vi "Write Create Tags_.vi"(8 "error in (no error)":errorcluster, 10 "Create Tags?":bool=TRUE, 11 "CVT configuration in":refnum<class "CVT configuration.lvclass">) -> (0 "error out":errorcluster, 3 "CVT configuration out":refnum<class "CVT configuration.lvclass">)   [LabVIEW 2013, in "CVT configuration.lvclass"]
uses:
  CVT configuration.lvclass
  CVT configuration.lvclass/CVT configuration.ctl
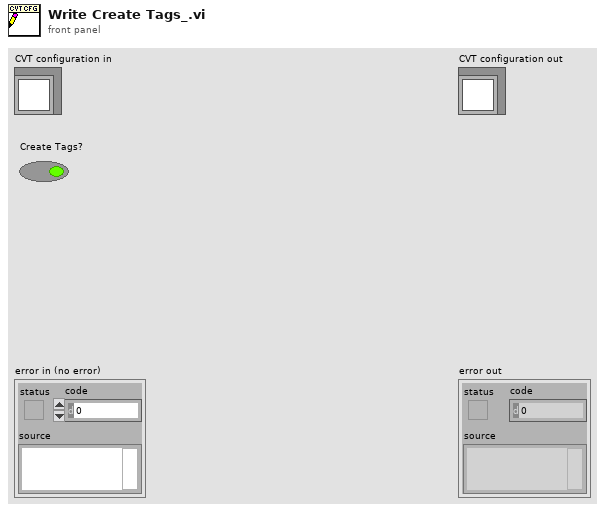
[diagram p1: front panel]
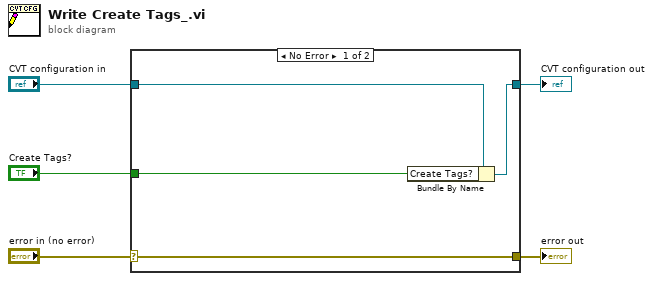
[diagram p0: block diagram]
diagram:
  n1 = case shown="No Error" "error in (no error)" {
    selector: "error in (no error)" -> [w9 w10]
    tunnel: [w9 w10] -> w4
    tunnel: [w7 w11] -> w2
    tunnel: "CVT configuration in" -> [w8 w11]
    tunnel: "Create Tags?" -> [w6 _]
    frame No Error {
      n2 = Bundle By Name(cluster=w8, "Create Tags?"=w6) -> (w7:refnum<class "CVT configuration.lvclass">)
    }
    frame Error {
    }
  }
  "error out" <- w4
  "CVT configuration out" <- w2
